vi "Loop_ACT_Shift.vi"   [LabVIEW 2017]
uses:
  ENUM_ACT_Solenoid_State.ctl
  <vilib>/Rock Robotics/WPI/Solenoid/WPI_SolenoidChannel.ctl
  ENUM_ACT_Solenoid_Action.ctl
  <vilib>/Rock Robotics/WPI/Solenoid/WPI_SolenoidValue.ctl
  <vilib>/Rock Robotics/WPI/Solenoid/WPI_SolenoidOpenDouble.vi
  _SHARE ALL/Global Share All/Global_STOP.vi
  Globals/Global_CMD_Gear.vi
  <vilib>/Rock Robotics/WPI/Solenoid/WPI_SolenoidSetEnum.vi
types:
  T1 = typedef "WPI_SolenoidChannel.ctl" = enum8{"Solenoid 0", "Solenoid 1", "Solenoid 2", "Solenoid 3", "Solenoid 4", "Solenoid 5", "Solenoid 6", "Solenoid 7", "Invalid"}
  T2 = typedef "ENUM_ACT_Solenoid_State.ctl" = enum16{"Startup", "Forward", "Reverse", "Idle", "Shutdown"}
  T3 = typedef "ENUM_ACT_Solenoid_Action.ctl" = enum16{"No Action", "Start", "Restart Timer", "Forward", "Reverse", "Off", "Close"}
  T4 = typedef "WPI_SolenoidDevRef.ctl" = cluster{"DevStatus":errorcluster, "Pneumatics Control Module":u8, "Forward Solenoid Channel":T1, "Reverse Solenoid Channel":T1}
  T5 = cluster{"State":T2, "Previous State":T2, "Current Time":timestamp, "Previous Time":timestamp, "Start Time":timestamp, "Target Time (ms)":u32, "Cycle Time(S)":dbl, "Solenoid In(T) Out(F)":bool, "SolenoidDevRef":T4}
  T6 = typedef "WPI_SolenoidValue.ctl" = enum16{"Off", "On", "Forward", "Reverse"}
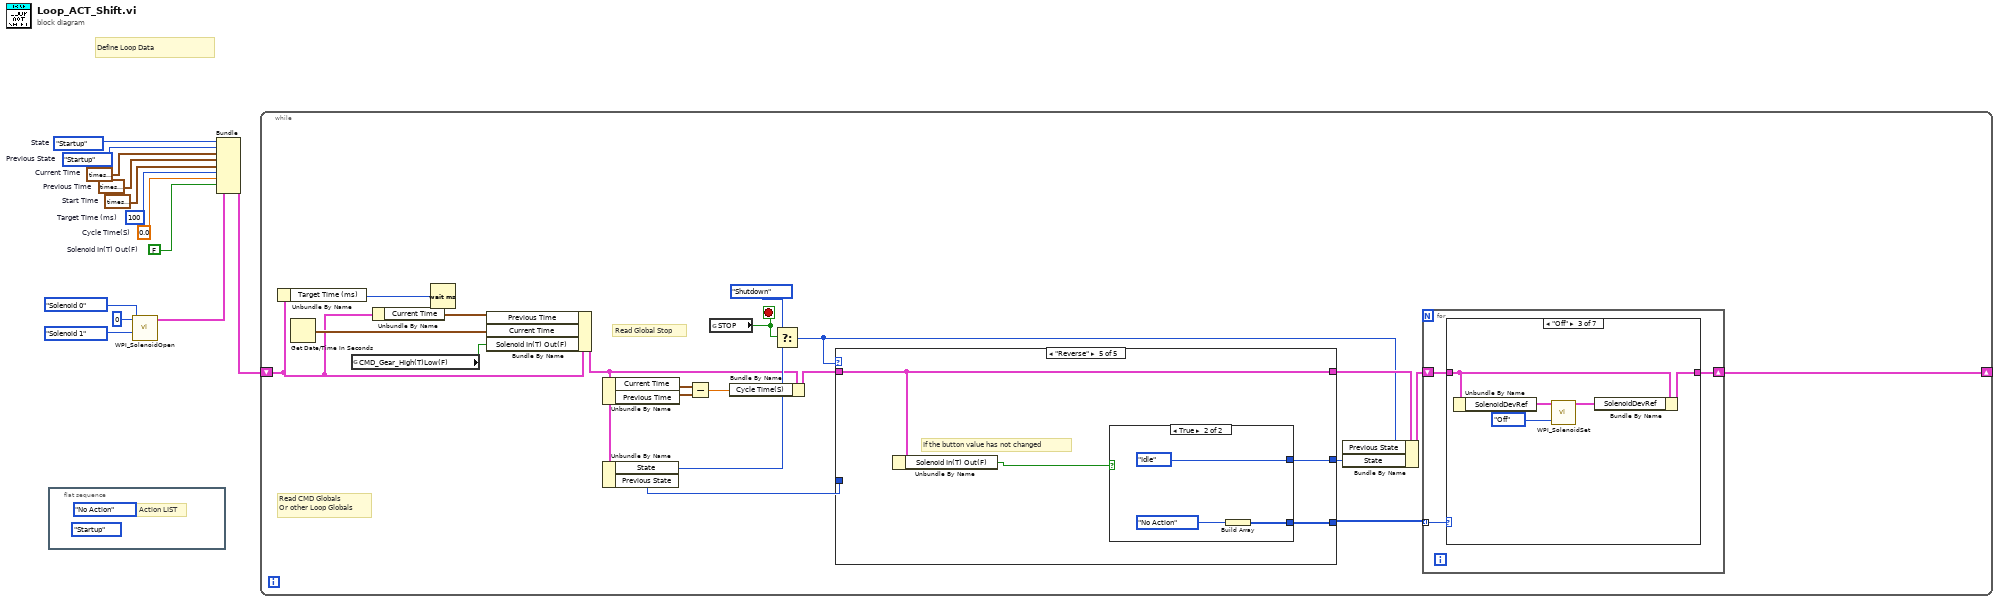
[diagram p0: block diagram]
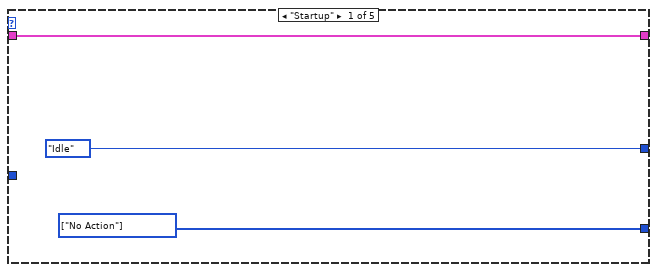
[diagram p2: hidden frame]
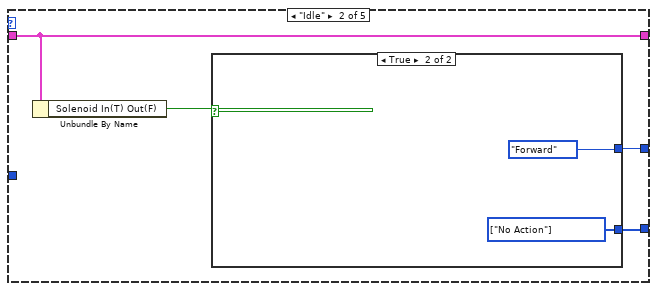
[diagram p3: hidden frame]
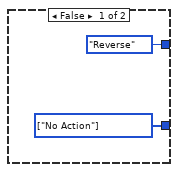
[diagram p4: hidden frame]
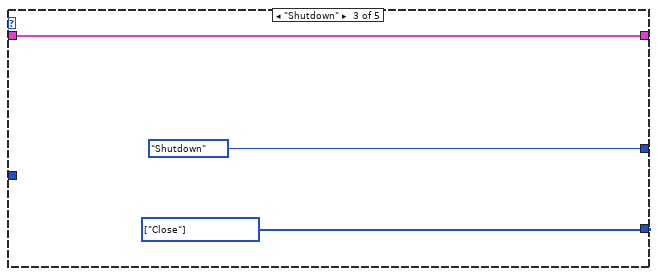
[diagram p5: hidden frame]
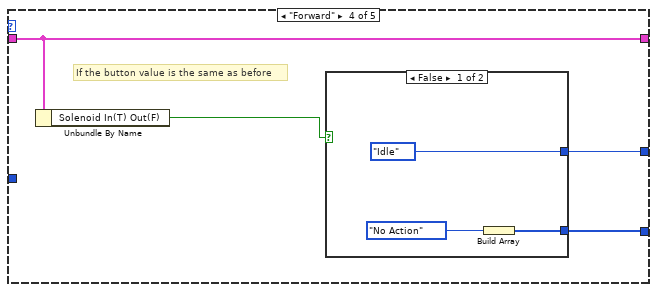
[diagram p6: hidden frame]
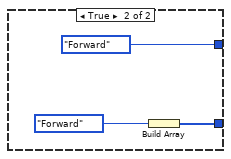
[diagram p7: hidden frame]
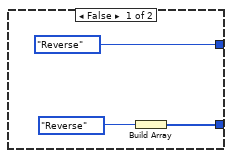
[diagram p8: hidden frame]
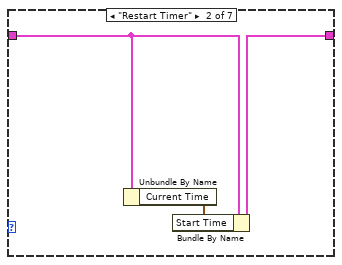
[diagram p10: hidden frame]
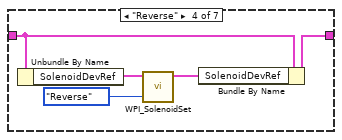
[diagram p11: hidden frame]
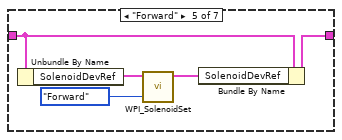
[diagram p12: hidden frame]
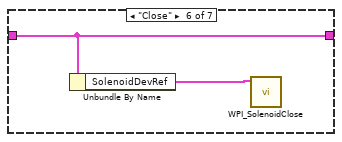
[diagram p13: hidden frame]
diagram:
  w5 = FALSE  # Solenoid In(T) Out(F)
  w6 = 0.0  # Cycle Time(S)
  w7 = ENUM_ACT_Solenoid_State."Startup"  # Previous State
  w8 = timestamp(0 s since 1904-01-01)  # Previous Time
  w9 = u32 100  # Target Time (ms)
  w10 = timestamp(0 s since 1904-01-01)  # Start Time
  w11 = timestamp(0 s since 1904-01-01)  # Current Time
  w12 = ENUM_ACT_Solenoid_State."Startup"  # State
  # "Define Loop Data"
  n1 = flat-sequence {
    frame #0 {
      (unwired) ENUM_ACT_Solenoid_State."Startup" ("State")
      (unwired) ENUM_ACT_Solenoid_Action."No Action" ("Action")
      # "Action LIST"
    }
  }
  n2 = call-poly <vilib>:"WPI_SolenoidOpen.vi"("Reverse Solenoid Channel"=WPI_SolenoidChannel."Solenoid 1", "Forward Solenoid Channel"=WPI_SolenoidChannel."Solenoid 0", "Pneumatics Control Module (0)"=u8 0) -> ("SolenoidDevRef"=w4:T4)  [unwired: 7 in, 1 out]
  n3 = Bundle("State"=w12, "Previous State"=w7, "Current Time"=w11, "Previous Time"=w8, "Start Time"=w10, "Target Time (ms)"=w9, "Cycle Time(S)"=w6, "Solenoid In(T) Out(F)"=w5, "SolenoidDevRef"=w4) -> (w13:T5)  [unwired: 1 in]
  n4 = while {
    shift-right: [w14] -> _
    shift-left: w13 -> [w24]
    stop <- w29 stop-if-true
    # "Read CMD Globals\nOr other Loop Globals"
    # "Read Global Stop"
    n5 = Unbundle By Name(w24) -> ("Target Time (ms)"=w26:u32)
    n6 = Get Date/Time In Seconds() -> (seconds since 1Jan1904=w33:timestamp)
    n7 = global read "Global_CMD_Gear.vi" "CMD_Gear_High(T)Low(F)"() -> (w16:bool)
    n8 = Unbundle By Name(w24) -> ("Current Time"=w25:timestamp)
    n9 = Wait (ms)(milliseconds to wait=w26) -> ()  [unwired: 1 out]
    n10 = Bundle By Name(cluster=w24, "Previous Time"=w25, "Current Time"=w33, "Solenoid In(T) Out(F)"=w16) -> (w20:T5)
    n11 = Unbundle By Name(w20) -> ("Current Time"=w21:timestamp, "Previous Time"=w22:timestamp)
    n12 = Unbundle By Name(w20) -> ("State"=w27:T2, "Previous State"=w23:T2)
    n13 = Subtract(x=w21, y=w22) -> (x-y=w18:dbl)
    n14 = global read "Global_STOP.vi" "STOP"() -> (w29:bool)
    n15 = Bundle By Name(cluster=w20, "Cycle Time(S)"=w18) -> (w19:T5)
    n16 = Select(t=ENUM_ACT_Solenoid_State."Shutdown" ("State"), s=w29, f=w27) -> (s? t:f=w15:T2)
    n17 = case shown="\"Reverse\"" w15 {
      tunnel: w19 -> [w36 w40 w47 w51 w59]
      tunnel: [w36 w40 w47 w51 w59] -> w31
      tunnel: [ENUM_ACT_Solenoid_State."Idle" ("State") w39 ENUM_ACT_Solenoid_State."Shutdown" ("State") w50 w61] -> w30
      tunnel: [w35 w38 w45 w49 w60] -> w17
      tunnel: w23 -> [_ _ _ _ _]
      frame "Startup" {
        w35 = T3[] [enum."No Action"] items=["No Action", "Start", "Restart Timer", "Forward", "Reverse", "Off", "Close"] ("Actions")
      }
      frame "Idle" {
        n18 = Unbundle By Name(w40) -> ("Solenoid In(T) Out(F)"=w37:bool)
        n19 = case shown="True" w37 {
          tunnel: [ENUM_ACT_Solenoid_State."Reverse" ("State") ENUM_ACT_Solenoid_State."Forward" ("State")] -> w39
          tunnel: [w41 w43] -> w38
          frame False {
            w41 = T3[] [enum."No Action"] items=["No Action", "Start", "Restart Timer", "Forward", "Reverse", "Off", "Close"]
          }
          frame True {
            w43 = T3[] [enum."No Action"] items=["No Action", "Start", "Restart Timer", "Forward", "Reverse", "Off", "Close"]
          }
        }
      }
      frame "Shutdown" {
        w45 = T3[] [enum."Close"] items=["No Action", "Start", "Restart Timer", "Forward", "Reverse", "Off", "Close"] ("Actions")
      }
      frame "Forward" {
        # "If the button value is the same as before"
        n20 = Unbundle By Name(w51) -> ("Solenoid In(T) Out(F)"=w48:bool)
        n21 = case shown="False" w48 {
          tunnel: [ENUM_ACT_Solenoid_State."Idle" ("State") ENUM_ACT_Solenoid_State."Forward" ("State")] -> w50
          tunnel: [w52 w56] -> w49
          frame False {
            n22 = Build Array(ENUM_ACT_Solenoid_Action."No Action" ("Action")) -> (w52:T3[])
          }
          frame True {
            n23 = Build Array(ENUM_ACT_Solenoid_Action."Forward" ("Action")) -> (w56:T3[])
          }
        }
      }
      frame "Reverse" {
        # "If the button value has not changed"
        n24 = Unbundle By Name(w59) -> ("Solenoid In(T) Out(F)"=w58:bool)
        n25 = case shown="True" w58 {
          tunnel: [ENUM_ACT_Solenoid_State."Reverse" ("State") ENUM_ACT_Solenoid_State."Idle" ("State")] -> w61
          tunnel: [w62 w66] -> w60
          frame False {
            n26 = Build Array(ENUM_ACT_Solenoid_Action."Reverse" ("Action")) -> (w62:T3[])
          }
          frame True {
            n27 = Build Array(ENUM_ACT_Solenoid_Action."No Action" ("Action")) -> (w66:T3[])
          }
        }
      }
    }
    n28 = Bundle By Name(cluster=w31, "Previous State"=w15, "State"=w30) -> (w32:T5)
    n29 = for {
      tunnel: w17 -> [w70] mode=indexing
      shift-right: [w69] -> w14
      shift-left: w32 -> [w68]
      n30 = case shown="\"Off\"" w70 {
        tunnel: w68 -> [w71 w74 w76 w81 w86 w90 w92]
        tunnel: [w71 w73 w75 w80 w85 w90 w92] -> w69
        frame "No Action" {
        }
        frame "Restart Timer" {
          n31 = Unbundle By Name(w74) -> ("Current Time"=w72:timestamp)
          n32 = Bundle By Name(cluster=w74, "Start Time"=w72) -> (w73:T5)
        }
        frame "Off" {
          n33 = Unbundle By Name(w76) -> ("SolenoidDevRef"=w79:T4)
          n34 = call-poly <vilib>:"WPI_SolenoidSet.vi"("Value"=WPI_SolenoidValue."Off", "SolenoidDevRef"=w79) -> ("SolenoidDevRef"=w77:T4)  [unwired: 8 in, 1 out]
          n35 = Bundle By Name(cluster=w76, "SolenoidDevRef"=w77) -> (w75:T5)
        }
        frame "Reverse" {
          n36 = Unbundle By Name(w81) -> ("SolenoidDevRef"=w84:T4)
          n37 = call-poly <vilib>:"WPI_SolenoidSet.vi"("Value"=WPI_SolenoidValue."Reverse", "SolenoidDevRef"=w84) -> ("SolenoidDevRef"=w82:T4)  [unwired: 8 in, 1 out]
          n38 = Bundle By Name(cluster=w81, "SolenoidDevRef"=w82) -> (w80:T5)
        }
        frame "Forward" {
          n39 = Unbundle By Name(w86) -> ("SolenoidDevRef"=w89:T4)
          n40 = call-poly <vilib>:"WPI_SolenoidSet.vi"("Value"=WPI_SolenoidValue."Forward", "SolenoidDevRef"=w89) -> ("SolenoidDevRef"=w87:T4)  [unwired: 8 in, 1 out]
          n41 = Bundle By Name(cluster=w86, "SolenoidDevRef"=w87) -> (w85:T5)
        }
        frame "Close" {
          n42 = Unbundle By Name(w90) -> ("SolenoidDevRef"=w91:T4)
          n43 = call <vilib>:"WPI_SolenoidClose.vi"("SolenoidDevRef"=w91) -> ()  [unwired: 10 in, 1 out]
        }
        frame "Start" {
        }
      }
    }
  }
